vi "Thumper Control.vi"(11 "Thump":bool) -> ()   [LabVIEW 2016]
uses:
  <vilib>/Rock Robotics/WPI/Solenoid/WPI_SolenoidSetEnum.vi
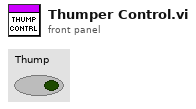
[diagram p1: front panel]
types:
  T1 = typedef "WPI_SolenoidDevRef.ctl" = cluster{"DevStatus":errorcluster, "Pneumatics Control Module":u8, "Forward Solenoid Channel":T2, "Reverse Solenoid Channel":T2}
  T2 = typedef "WPI_SolenoidChannel.ctl" = enum8{"Solenoid 0", "Solenoid 1", "Solenoid 2", "Solenoid 3", "Solenoid 4", "Solenoid 5", "Solenoid 6", "Solenoid 7", "Invalid"}
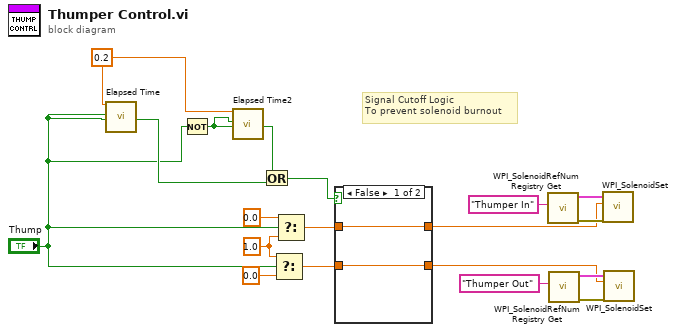
[diagram p0: block diagram]
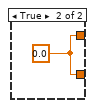
[diagram p2: hidden frame]
diagram:
  w13 = 0.2 ("Time Target (s)")
  w8 = 1.0 ("f")
  # "Signal Cutoff Logic\nTo prevent solenoid burnout"
  n1 = call "Elapsed Time"("Time Target (s)"=w13, "Reset"="Thump", "Auto Reset"="Thump") -> ("Time has Elapsed"=w10:bool)  [unwired: 9 in, 7 out]
  n2 = Not(x="Thump") -> (.not. x?=w12:bool)
  n3 = call "Elapsed Time2"("Time Target (s)"=w13, "Reset"=w12, "Auto Reset"=w12) -> ("Time has Elapsed"=w11:bool)  [unwired: 9 in, 7 out]
  n4 = Or(x=w11, y=w10) -> (x .or. y?=w9:bool)
  n5 = Select(t=w8, s="Thump", f=0.0) -> (s? t:f=w6:dbl)
  n6 = Select(t=0.0, s="Thump", f=w8) -> (s? t:f=w4:dbl)
  n7 = case shown="False" w9 {
    tunnel: [w21 w22] -> w7
    tunnel: w6 -> [w21 _]
    tunnel: [w20 w22] -> w5
    tunnel: w4 -> [w20 _]
    frame False {
    }
    frame True {
      w22 = 0.0 ("f")
    }
  }
  n8 = call <vilib>:"WPI_SolenoidRefNum Registry Get.vi"("refnum name"="Thumper In") -> ("error out"=w19:errorcluster, "SolenoidDevRef"=w18:T1)  [unwired: 9 in]
  n9 = call <vilib>:"WPI_SolenoidRefNum Registry Get.vi"("refnum name"="Thumper Out") -> ("error out"=w16:errorcluster, "SolenoidDevRef"=w15:T1)  [unwired: 9 in]
  n10 = call-poly <vilib>:"WPI_SolenoidSet.vi"("error in (no error)"=w19, "Value"=w5, "SolenoidDevRef"=w18) -> ()  [unwired: 7 in, 2 out]
  n11 = call-poly <vilib>:"WPI_SolenoidSet.vi"("error in (no error)"=w16, "Value"=w7, "SolenoidDevRef"=w15) -> ()  [unwired: 7 in, 2 out]
